vi "Team072 FinalDemo.vi"   [LabVIEW 2016]
uses:
  <vilib>/NXT/Block Support/NXT_InputPort.ctl
  <vilib>/NXT/Subs/MotorOutput.ctl
  <vilib>/NXT/Dual Mode Library/Sensors/Light_On.vi
  <vilib>/NXT/Dual Mode Library/Motors/MotorOn.vi
  <vilib>/NXT/Dual Mode Library/Waits/Wait_Num(msec).vi
types:
  T1 = typedef "NXT_InputPort.ctl" = u32
  T2 = typedef "MotorOutput.ctl" = u8
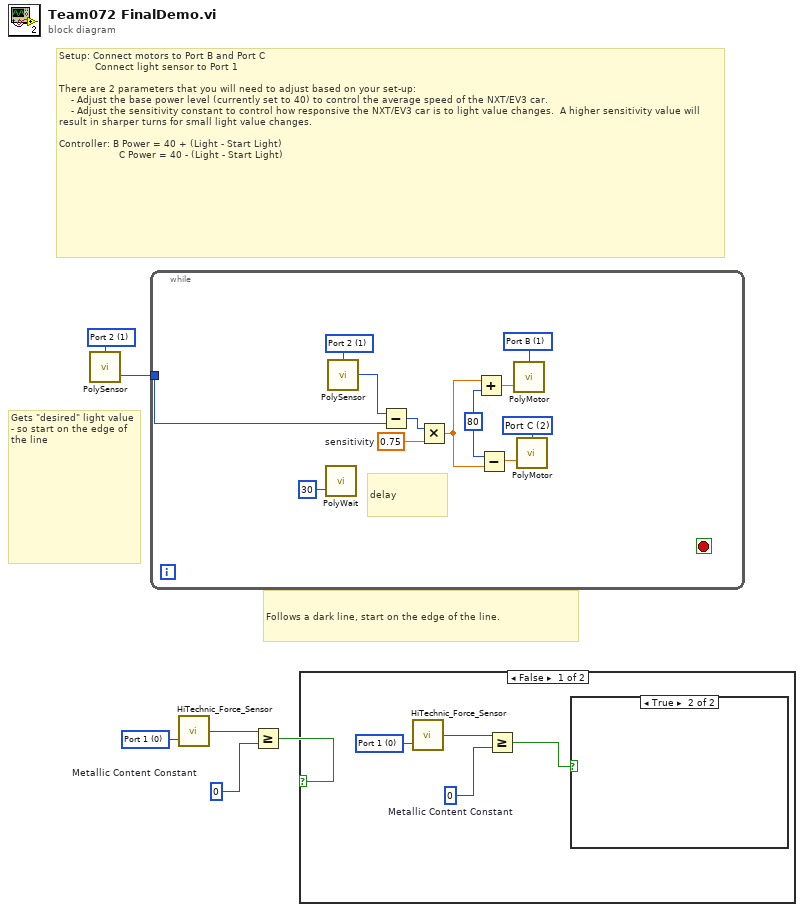
[diagram p0: block diagram]
diagram:
  w2 = i16 0  # Metallic Content Constant
  w4 = T1 0 items=["Port 1", "Port 2", "Port 3", "Port 4"] ("Port (Port 1)")
  w5 = T1 1 items=["Port 1", "Port 2", "Port 3", "Port 4"] ("Input Port (Port 3)")
  # "Gets \"desired\" light value - so start on the edge of the line"
  # "Follows a dark line, start on the edge of the line."
  # "Setup: Connect motors to Port B and Port C\n            Connect light sensor to Port 1\n\nThere are 2 parameters that you will need to adjust based on your set-up:  \n    - Adjust the base power level (currently set to 40) to control the average speed of the NXT/EV3 car.\n    - Adjust the sensitivity constant to control how responsive the NXT/EV3 car is to light value changes.  A higher sensitivity value will result in sharper turns for small light value changes. \n \nController: B Power = 40 + (Light - Start Light)\n                    C Power = 40 - (Light - Start Light)"
  n1 = call-poly <vilib>:"PolySensor.vi"("Port (Port 3)"=w5) -> ("Scaled Value"=w6:i16)  [unwired: 1 in, 2 out]
  n2 = while {
    tunnel: w6 -> [w13]
    stop <- _ stop-if-true
    w7 = T2 2 items=["Port A"=0, "Port B"=1, "Port C"=2, "Ports A & B"=4, "Ports A & C"=5, "Ports B & C"=6, "All Ports"=3] ("Output Port (All Ports)")
    w8 = T2 1 items=["Port A"=0, "Port B"=1, "Port C"=2, "Ports A & B"=4, "Ports A & C"=5, "Ports B & C"=6, "All Ports"=3] ("Output Port (All Ports)")
    w9 = sgl 0.75  # sensitivity
    w15 = 80 ("y")
    w18 = T1 1 items=["Port 1", "Port 2", "Port 3", "Port 4"] ("Input Port (Port 3)")
    # "delay"
    n3 = call-poly <vilib>:"PolyWait.vi"("Time (100 msec)"=u32 30 ("Time (1 sec)")) -> ()  [unwired: 3 in, 1 out]
    n4 = call-poly <vilib>:"PolySensor.vi"("Port (Port 3)"=w18) -> ("Scaled Value"=w17:i16)  [unwired: 1 in, 2 out]
    n5 = Subtract(x=w17, y=w13) -> (x-y=w11:i16)
    n6 = Multiply(x=w11, y=w9) -> (x*y=w10:sgl)
    n7 = Add(x=w10, y=w15) -> (x+y=w16:sgl)
    n8 = Subtract(x=w15, y=w10) -> (x-y=w14:sgl)
    n9 = call-poly <vilib>:"PolyMotor.vi"("Power (75)"=w16, "Output Port (All Ports)"=w8) -> ()  [unwired: 1 in, 2 out]
    n10 = call-poly <vilib>:"PolyMotor.vi"("Power (75)"=w14, "Output Port (All Ports)"=w7) -> ()  [unwired: 1 in, 2 out]
  }
  n11 = call "HiTechnic_Force_Sensor.vi"("Port (Port 1)"=w4) -> ("Scaled Value"=w3:i16)  [unwired: 1 in, 2 out]
  n12 = Greater Or Equal?(x=w3, y=w2) -> (x >= y?=w1:bool)
  n13 = case shown="False" w1 {
    frame False {
      w20 = i16 0  # Metallic Content Constant
      w22 = T1 0 items=["Port 1", "Port 2", "Port 3", "Port 4"] ("Port (Port 1)")
      n14 = call "HiTechnic_Force_Sensor.vi"("Port (Port 1)"=w22) -> ("Scaled Value"=w21:i16)  [unwired: 1 in, 2 out]
      n15 = Greater Or Equal?(x=w21, y=w20) -> (x >= y?=w19:bool)
      n16 = case shown="True" w19 {
        frame False {
        }
        frame True {
        }
      }
    }
    frame True {
    }
  }
